vi "Add MB Address.vi"(8 "error in (no error)":errorcluster, 10 "Starting Address (SGL) in":i32, 11 "Channel in":refnum<class "Channel.lvclass">) -> (0 "error out":errorcluster, 2 "Next Address (SGL)":i32, 3 "Channel out":refnum<class "Channel.lvclass">)   [LabVIEW 2012, in "Measurement Channels.lvlib" / "Channel.lvclass"]
uses:
  Channel.lvclass
  Channel.lvclass/Channel.ctl
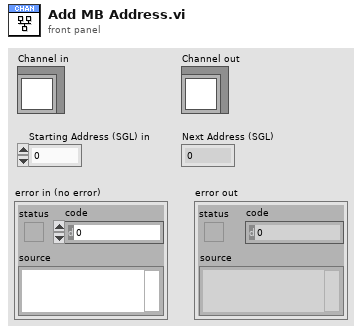
[diagram p1: front panel]
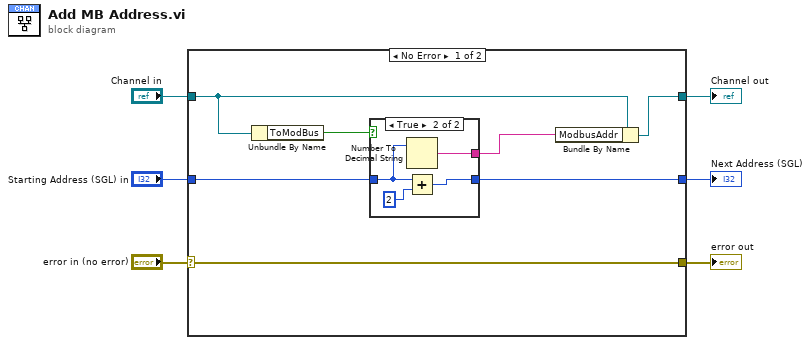
[diagram p0: block diagram]
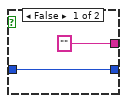
[diagram p2: hidden frame]
diagram:
  n1 = case shown="No Error" "error in (no error)" {
    selector: "error in (no error)" -> [w7 w20]
    tunnel: "Starting Address (SGL) in" -> [w13 w21]
    tunnel: [w12 w21] -> w5
    tunnel: "Channel in" -> [w10 w22]
    tunnel: [w9 w22] -> w3
    tunnel: [w7 w20] -> w1
    frame No Error {
      n2 = Unbundle By Name(w10) -> ("ToModBus"=w11:bool)
      n3 = case shown="True" w11 {
        tunnel: [w15 w19] -> w12
        tunnel: w13 -> [w15 w17]
        tunnel: ["" ("ModbusAddr") w16] -> w8
        frame False {
        }
        frame True {
          n4 = Number To Decimal String(number=w17) -> (decimal integer string=w16:string)  [unwired: 1 in]
          n5 = Add(x=w17, y=2) -> (x+y=w19:i32)
        }
      }
      n6 = Bundle By Name(cluster=w10, "ModbusAddr"=w8) -> (w9:refnum<class "Channel.lvclass">)
    }
    frame Error {
    }
  }
  "Channel out" <- w3
  "Next Address (SGL)" <- w5
  "error out" <- w1
